vi "FetchVal34980awh.vi"(0 "connection ID In":refnum<k5>, 7 "Circuit ID":i32=1016 format="%_4g", 11 "error in (no error)":errorcluster) -> (4 "connection ID Out":refnum<k5>, 8 "Value":dbl format="%#_10e", 15 "Error out":errorcluster)   [LabVIEW 2009]
doc: "Reads a value from the 34980. \nAssumes that you have scanned the 34980 to store the values."
panel:
  # "This assumes you have already scanned the 34980"
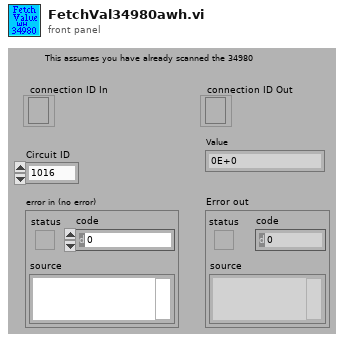
[diagram p1: front panel]
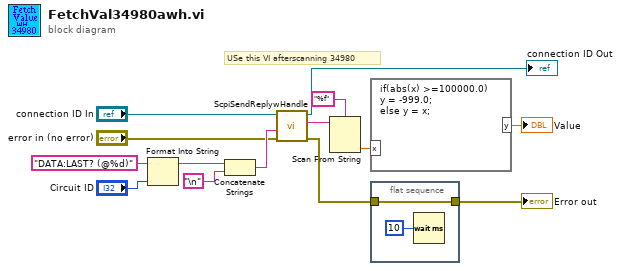
[diagram p0: block diagram]
diagram:
  # "USe this VI afterscanning 34980"
  n1 = Format Into String(format string="DATA:LAST? (@%d)", "Circuit ID") -> (resulting string=w11:string)  [unwired: 2 in, 1 out]
  n2 = Concatenate Strings(w11, "\n") -> (w7:string)
  n3 = call "ScpiSendReplywHandle.vi"("error in (no error)"="error in (no error)", "Command"=w7, "connection ID In"="connection ID In") -> ("Error out"=w3:errorcluster, "Reply"=w4:string, "connection ID Out"=→"connection ID Out":refnum<k5>)  [unwired: 5 in]
  n4 = Scan From String(format string="%f", input string=w4) -> (output 1=w9:dbl)  [unwired: 3 in, 3 out]
  n5 = formula code="if(abs(x) >=100000.0)\ny = -999.0;\nelse y = x;"("x"=w9) -> ("y"=→"Value":dbl)
  n6 = flat-sequence {
    tunnel: w3 -> [w15]
    tunnel: [w15] -> w2
    frame #0 {
      n7 = Wait (ms)(milliseconds to wait=u32 10) -> ()  [unwired: 1 out]
    }
  }
  "Error out" <- w2
